vi "InsidelHandle_1.vi"(7 "Mode":enum16{"Open", "Read", "Write", "Close"}(ring), 8 "error in (no error)":errorcluster, 9 "data in":string, 10 "Port":u16=6342, 11 "Machine":string="localhost") -> (0 "error out":errorcluster, 1 "data out":string)   [LabVIEW 2011]
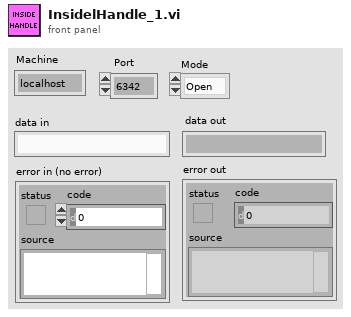
[diagram p1: front panel]
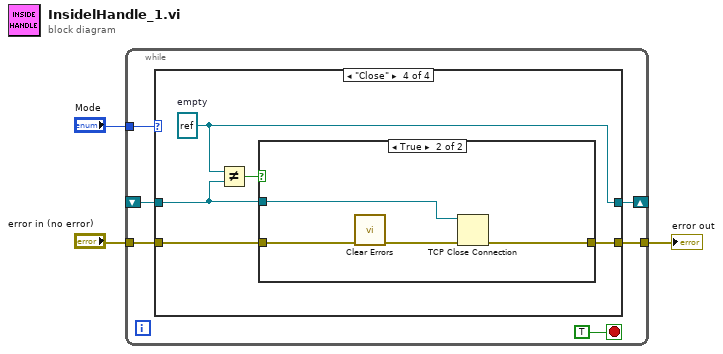
[diagram p0: block diagram]
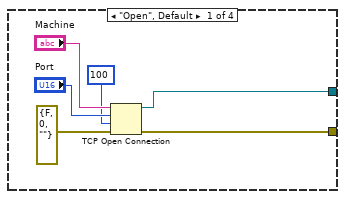
[diagram p2: hidden frame]
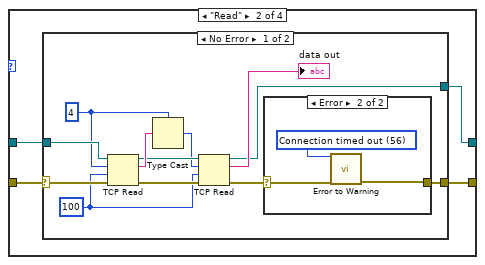
[diagram p3: hidden frame]
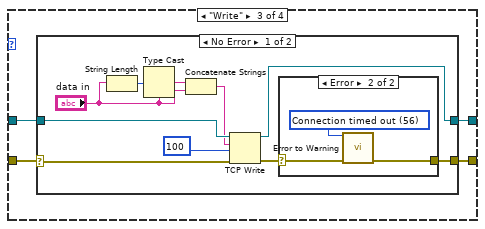
[diagram p6: hidden frame]
diagram:
  n1 = while {
    shift-right: [w9] -> _
    shift-left: _ -> [w6]
    tunnel: "Mode" -> [w5]
    tunnel: "error in (no error)" -> [w7]
    tunnel: [w8] -> w1
    stop <- TRUE stop-if-true
    n2 = case shown="\"Close\"" w5 {
      tunnel: [w12 w18 w40 w59] -> w9
      tunnel: [w10 w16 w39 w62] -> w8
      tunnel: w7 -> [_ w17 w38 w61]
      tunnel: w6 -> [_ w19 w41 w58]
      frame "Open", Default {
        n3 = TCP Open Connection(address="Machine", remote port or service name="Port", timeout ms (60000)=100, error in (no error)=errorcluster {"status"=FALSE, "code"=0, "source"=""} ("error constant")) -> (connection ID=w12:refnum<k5>, error out=w10:errorcluster)  [unwired: 1 out]
      }
      frame "Read" {
        n4 = case shown="No Error" w17 {
          selector: w17 -> [w30 w36]
          tunnel: w19 -> [w31 w37]
          tunnel: [w21 w37] -> w18
          tunnel: [w29 w36] -> w16
          frame No Error {
            w23 = 100
            w24 = 4 ("bytes to read")
            n5 = TCP Read(connection ID=w31, bytes to read=w24, error in (no error)=w30, 9:w23) -> (connection ID out=w26:refnum<k5>, data out=w27:string, error out=w28:errorcluster)  [unwired: 1 out]
            n6 = Type Cast(type=w24, x=w27) -> (*(type *) &x=w25:i32)
            n7 = TCP Read(connection ID=w26, bytes to read=w25, error in (no error)=w28, 9:w23) -> (connection ID out=w21:refnum<k5>, data out=→"data out":string, error out=w20:errorcluster)  [unwired: 1 out]
            n8 = case shown="Error" w20 {
              selector: w20 -> [w32 w35]
              tunnel: [w32 w33] -> w29
              frame No Error {
              }
              frame Error {
                w34 = 56 items=["No Error", "Argument Error", "Memory Full", "Out of Zone", "End of File", "File Already Open", "Generic File IO Error", "File Not Found", "File Permission Error", "Disk Full", "Duplicate Path", "Too Many Files Open", "Not Enabled", "Resource File Not Found", "Cannot Add Resource", "Resource Not Found", "Image Not Found", "Image Memory Error", "Pen Does Not Exist", "Config Bad Type", "Config Token Not Found", "Config Parse Error", "Config Memory Error", "Bad External Code Format", "Bad External Code Offset", "External Code Not Present", "Null Window", "Destroy Window Mixup", "Null Menu", "Print Aborted", "Bad Print Record", "Print Driver Error", "Windows Error During Print", "Memory Error During Print", "Print Dialog Error", "Generic Print Error", "Invalid Device Refnum", "Device Not Found", "Device Parameter Error", "Device Unit Error", "Can't Open Device", "Device Call Aborted", "Generic Error", "Cancelled By User", "Object ID Too Low", "Object ID Too High", "Object Not In Heap", "Unknown Heap", "Bad DefProc ID", "DefProc Not In Table", "Message Out Of Range", "Null Method", "Unknown Message", "Manager Call Not Supported", "Bad address", "Connection In progress", "Connection timed out", "Connection is already in progress", "Network attribute not supported", "Network error", "Address in use", "System out of memory", "Connection aborted", "Connection refused", "Connection is not connected", "Connection is already connected", "Connection closed", "Initialize error (interapplication manager)", "Bad occurrence", "Wait on unbound occurrence handler", "Occurrence queue overflow", "Bad path", "Semaphore not signaled", "Unrecognized type (interapplication manager)"] ("1st Error to Convert")
                n9 = call <vilib>:"Error to Warning.vi"("1st Error to Convert"=w34, "error in"=w35) -> ("warning out"=w33:errorcluster)  [unwired: 3 in, 10 out]
              }
            }
          }
          frame Error {
          }
        }
      }
      frame "Write" {
        n10 = case shown="No Error" w38 {
          selector: w38 -> [w48 w56]
          tunnel: w41 -> [w51 w57]
          tunnel: [w42 w57] -> w40
          tunnel: [w49 w56] -> w39
          frame No Error {
            n11 = String Length(string="data in") -> (length=w46:i32)
            n12 = Type Cast(type="data in", x=w46) -> (*(type *) &x=w47:string)
            n13 = Concatenate Strings(w47, "data in") -> (w44:string)
            n14 = TCP Write(connection ID=w51, data in=w44, error in (no error)=w48, 9:100 ("timeout ms (25000)")) -> (connection ID out=w42:refnum<k5>, error out=w43:errorcluster)  [unwired: 1 out]
            n15 = case shown="Error" w43 {
              selector: w43 -> [w52 w53]
              tunnel: [w52 w54] -> w49
              frame No Error {
              }
              frame Error {
                w55 = 56 items=["No Error", "Argument Error", "Memory Full", "Out of Zone", "End of File", "File Already Open", "Generic File IO Error", "File Not Found", "File Permission Error", "Disk Full", "Duplicate Path", "Too Many Files Open", "Not Enabled", "Resource File Not Found", "Cannot Add Resource", "Resource Not Found", "Image Not Found", "Image Memory Error", "Pen Does Not Exist", "Config Bad Type", "Config Token Not Found", "Config Parse Error", "Config Memory Error", "Bad External Code Format", "Bad External Code Offset", "External Code Not Present", "Null Window", "Destroy Window Mixup", "Null Menu", "Print Aborted", "Bad Print Record", "Print Driver Error", "Windows Error During Print", "Memory Error During Print", "Print Dialog Error", "Generic Print Error", "Invalid Device Refnum", "Device Not Found", "Device Parameter Error", "Device Unit Error", "Can't Open Device", "Device Call Aborted", "Generic Error", "Cancelled By User", "Object ID Too Low", "Object ID Too High", "Object Not In Heap", "Unknown Heap", "Bad DefProc ID", "DefProc Not In Table", "Message Out Of Range", "Null Method", "Unknown Message", "Manager Call Not Supported", "Bad address", "Connection In progress", "Connection timed out", "Connection is already in progress", "Network attribute not supported", "Network error", "Address in use", "System out of memory", "Connection aborted", "Connection refused", "Connection is not connected", "Connection is already connected", "Connection closed", "Initialize error (interapplication manager)", "Bad occurrence", "Wait on unbound occurrence handler", "Occurrence queue overflow", "Bad path", "Semaphore not signaled", "Unrecognized type (interapplication manager)"] ("1st Error to Convert")
                n16 = call <vilib>:"Error to Warning.vi"("1st Error to Convert"=w55, "error in"=w53) -> ("warning out"=w54:errorcluster)  [unwired: 3 in, 10 out]
              }
            }
          }
          frame Error {
          }
        }
      }
      frame "Close" {
        w59 = refnum<k5> refnum  # empty
        n17 = Not Equal?(x=w59, y=w58) -> (x != y?=w60:bool)
        n18 = case shown="True" w60 {
          tunnel: [w63 w67] -> w62
          tunnel: w61 -> [w63 w66]
          tunnel: w58 -> [_ w64]
          frame False {
          }
          frame True {
            n19 = call <vilib>:"Clear Errors.vi"("error in (no error)"=w66) -> ("error out"=w65:errorcluster)  [unwired: 6 in]
            n20 = TCP Close Connection(connection ID=w64, error in (no error)=w65) -> (error out=w67:errorcluster)  [unwired: 2 out]
          }
        }
      }
    }
  }
  "error out" <- w1
